vi "AssertAllItems.vi"(0 "VI Reference In":refnum<vi>, 1 "Test Label":string, 2 "delimiter (>>)":string=">>", 3 "Assert Only? (F)":bool, 5 "Control Path":string, 7 "Item Value":string[][](array[string]), 11 "Error In":errorcluster, 12 "Assert Interval(10 ms)":u32=10, 13 "Timeout(5 sec)":dbl=5.0) -> (4 "VI Reference Out":refnum<vi>, 6 "Asserted Value":string[][](array[string]), 15 "Error Out":errorcluster)   [LabVIEW 2016, in "Drona.lvlib" / "AssertControlValue.lvlib" / "AssertTable.lvlib"]
doc: "Asserts if the items in the table control is equal.\n\nThe input control name is given as a string , incase of path, use delimiters inbetween the path.\nThis VI gets the value of the control, untill the value is equal to the input value."
uses:
  AssertTable.lvlib
  Get/GetControlRef/GetControlRefByPath.vi
  <vilib>/addons/_JKI Toolkits/Caraya/classes/Assert/Assert Equal Value_Variant.vi
  <vilib>/Utility/error.llb/Error Cluster From Error Code.vi
  <vilib>/ErrorRing/Error Ring.xnode
  Get/GetControlRef/GetControlRef.lvlib
  <vilib>/addons/_JKI Toolkits/Caraya/classes/Assert/Assert.lvclass
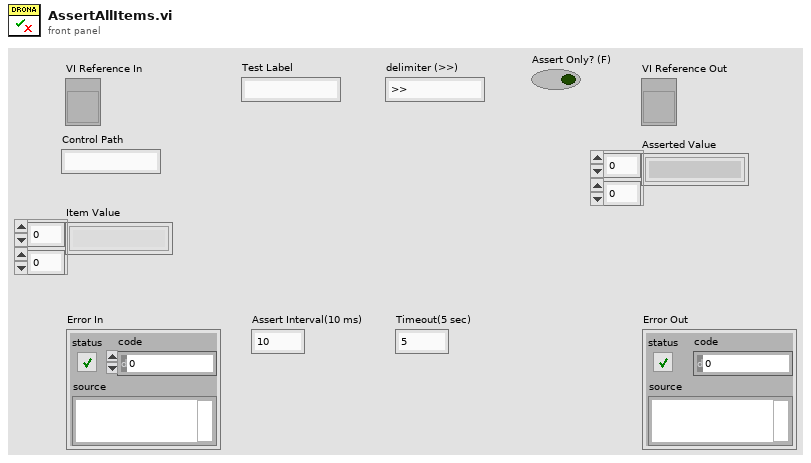
[diagram p1: front panel]
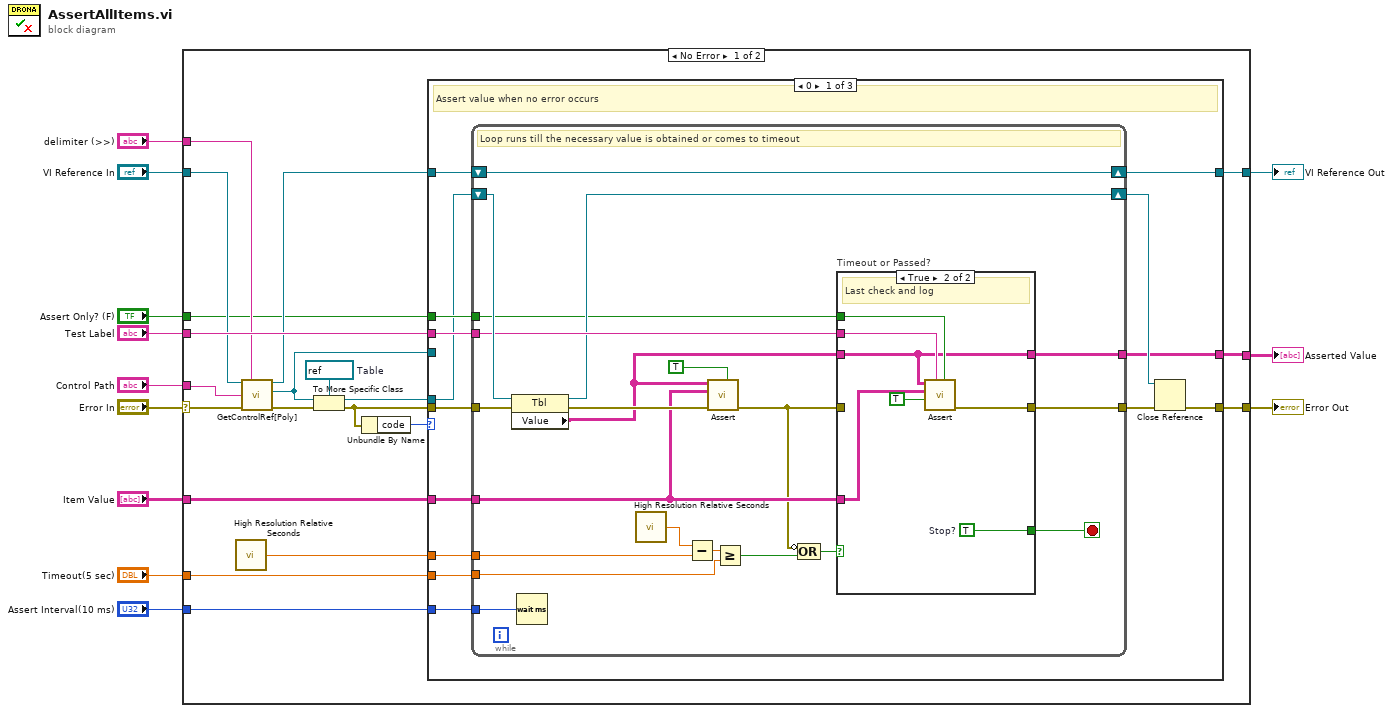
[diagram p0: block diagram]
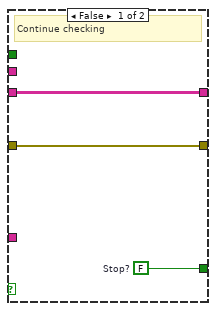
[diagram p2: hidden frame]
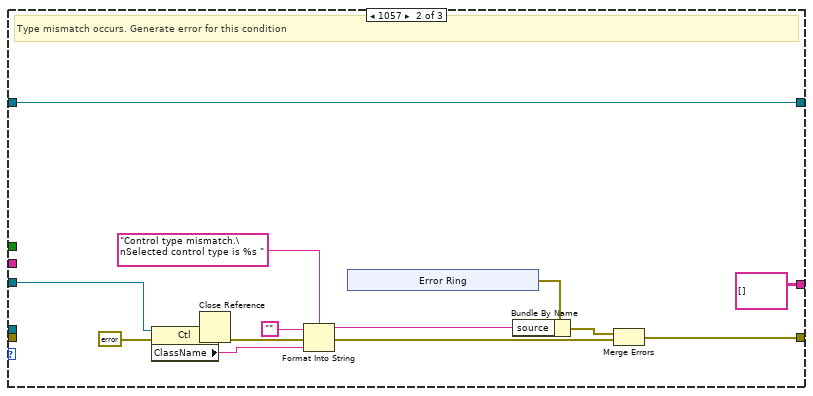
[diagram p3: hidden frame]
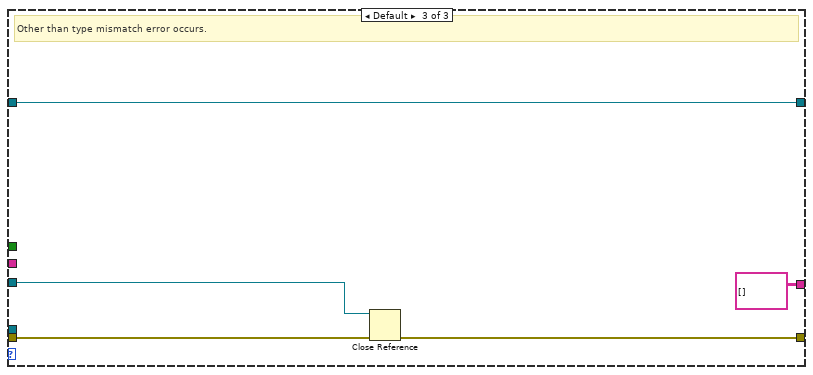
[diagram p4: hidden frame]
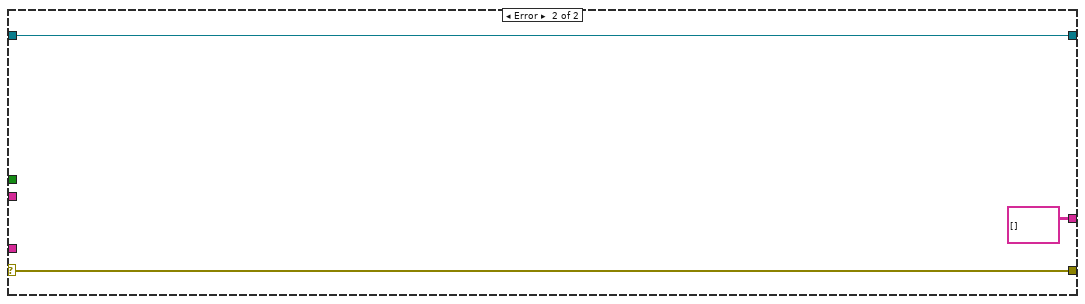
[diagram p5: hidden frame]
diagram:
  n1 = case shown="No Error" "Error In" {
    selector: "Error In" -> [w28 w105]
    tunnel: "Timeout(5 sec)" -> [w32 _]
    tunnel: [w31 w104] -> w11
    tunnel: [w22 w105] -> w10
    tunnel: "Assert Interval(10 ms)" -> [w30 _]
    tunnel: "Test Label" -> [w29 _]
    tunnel: "VI Reference In" -> [w27 w104]
    tunnel: "Control Path" -> [w26 _]
    tunnel: "delimiter (>>)" -> [w21 _]
    tunnel: "Assert Only? (F)" -> [w20 _]
    tunnel: [w19 string[][] [] ("Value")] -> w1
    tunnel: "Item Value" -> [w16 _]
    frame No Error {
      w18 = refnum<vi> refnum  # Table
      n2 = call <vilib>:"High Resolution Relative Seconds.vi"() -> ("relative seconds"=w25:dbl)
      n3 = call-poly "GetControlRef[Poly].vi"("VI Reference In"=w27, "delimiter (>>)"=w21, "Control Path"=w26, "error In"=w28) -> ("VI Reference Out"=w23:refnum<vi>, "Ctl Refnum"=w13:refnum<vi>, "error out"=w24:errorcluster)  [unwired: 9 in]
      n4 = To More Specific Class(target class=w18, reference=w13, error in=w24) -> (specific class reference=w17:refnum<vi>, error out=w15:errorcluster)
      n5 = Unbundle By Name(w15) -> ("code"=w14:i32)
      n6 = case shown="0" w14 {
        tunnel: w32 -> [w46 _ _]
        tunnel: [w45 w92 w102] -> w31
        tunnel: w30 -> [w43 _ _]
        tunnel: w29 -> [w42 _ _]
        tunnel: w25 -> [w41 _ _]
        tunnel: w23 -> [w40 w92 w102]
        tunnel: [w39 w80 w100] -> w22
        tunnel: w20 -> [w37 _ _]
        tunnel: [w36 string[][] [] ("Value") string[][] [] ("Value")] -> w19
        tunnel: w15 -> [w35 _ w101]
        tunnel: w17 -> [w34 _ _]
        tunnel: w16 -> [w33 _ _]
        tunnel: w13 -> [_ w79 w99]
        frame 0 {
          # "Assert value when no error occurs"
          n7 = while {
            tunnel: w46 -> [w66]
            tunnel: w41 -> [w67]
            tunnel: w35 -> [w61]
            tunnel: [w64] -> w44
            tunnel: w43 -> [w62]
            tunnel: w42 -> [w58]
            shift-right: [w59] -> w45
            shift-left: w40 -> [w59]
            shift-right: [w57] -> w38
            shift-left: w34 -> [w60]
            tunnel: w37 -> [w56]
            tunnel: [w55] -> w36
            tunnel: w33 -> [w54]
            stop <- w65 stop-if-true
            # "Loop runs till the necessary value is obtained or comes to timeout"
            n8 = property on="Property Node" class="Tbl"(reference=w60, error in=w61) -> (reference out=w57:refnum<vi>, error out=w63:errorcluster, "Value"=w47:string[][])
            n9 = Wait (ms)(milliseconds to wait=w62) -> ()  [unwired: 1 out]
            n10 = call <vilib>:"High Resolution Relative Seconds.vi"() -> ("relative seconds"=w53:dbl)
            n11 = Subtract(x=w53, y=w67) -> (x-y=w52:dbl)
            n12 = call-poly <vilib>:"Assert.vi"("Assert Only? (F)"=TRUE, "error in (no error)"=w63, "Y"=w54, "X"=w47) -> ("error out"=w50:errorcluster)  [unwired: 6 in, 1 out]
            n13 = Greater Or Equal?(x=w52, y=w66) -> (x >= y?=w51:bool)
            n14 = Compound Arithmetic op=OR(invert w50, w51) -> (w49:bool)
            n15 = case "Timeout or Passed?" shown="True" w49 {
              tunnel: w50 -> [w70 _]
              tunnel: w54 -> [_ w76]
              tunnel: w47 -> [w68 w71]
              tunnel: w58 -> [_ w77]
              tunnel: [w70 w75] -> w64
              tunnel: [w69 w74] -> w65
              tunnel: w56 -> [_ w72]
              tunnel: [w68 w71] -> w55
              frame False {
                w69 = FALSE  # Stop?
                # "Continue checking"
              }
              frame True {
                w74 = TRUE  # Stop?
                # "Last check and log"
                n16 = call-poly <vilib>:"Assert.vi"("Assert Only? (F)"=w72, "Label"=w77, "Register with caller test (F)"=TRUE, "Y"=w76, "X"=w71) -> ("error out"=w75:errorcluster)  [unwired: 5 in, 1 out]
              }
            }
          }
          n17 = Close Reference(reference=w38, error in (no error)=w44) -> (error out=w39:errorcluster)
        }
        frame 1057 {
          # "Type mismatch occurs. Generate error for this condition"
          n18 = property class="Ctl"(reference=w79, error in=errorcluster {"status"=FALSE, "code"=0, "source"=""} ("error out")) -> (reference out=w81:refnum<vi>, error out=w91:errorcluster, "ClassName"=w88:string)
          n19 = Close Reference(reference=w81, error in (no error)=w91) -> (error out=w82:errorcluster)
          n20 = Format Into String(format string="Control type mismatch.\nSelected control type is %s ", initial string="", error in=w82, w88) -> (resulting string=w85:string, error out=w83:errorcluster)
          n21 = xnode "Error Ring"() -> ("error out"=w86:errorcluster)
          n22 = Bundle By Name(cluster=w86, "source"=w85) -> (w84:errorcluster)
          n23 = Merge Errors(w84, w83) -> (w80:errorcluster)
        }
        frame Default {
          # "Other than type mismatch error occurs."
          n24 = Close Reference(reference=w99, error in (no error)=w101) -> (error out=w100:errorcluster)
        }
      }
    }
    frame Error {
    }
  }
  "Error Out" <- w10
  "VI Reference Out" <- w11
  "Asserted Value" <- w1
